vi "Initialize Weather Station.vi"(8 "error in (no error)":errorcluster) -> (0 "error out":errorcluster, 3 "file refnum":refnum<file>, 5 "Weather Data":T1)   [LabVIEW 2010]
doc: "This VI is a part of the Weather Station project. The weather data cluster is created, and a text file (Weather.txt) is created. A header representing the weather data cluster is written to the file.\n\nInputs: Error In\nOutputs: File Refnum, Weather Data Cluster, Error Out"
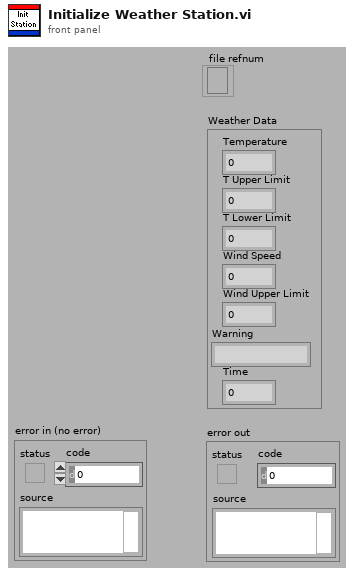
[diagram p1: front panel]
types:
  T1 = cluster{"Temperature":dbl, "T Upper Limit":dbl, "T Lower Limit":dbl, "Wind Speed":dbl, "Wind Upper Limit":dbl, "Warning":string, "Time":dbl}
  T2 = enum16{"open", "replace", "create", "open or create", "replace or create", "replace or create with confirmation"}
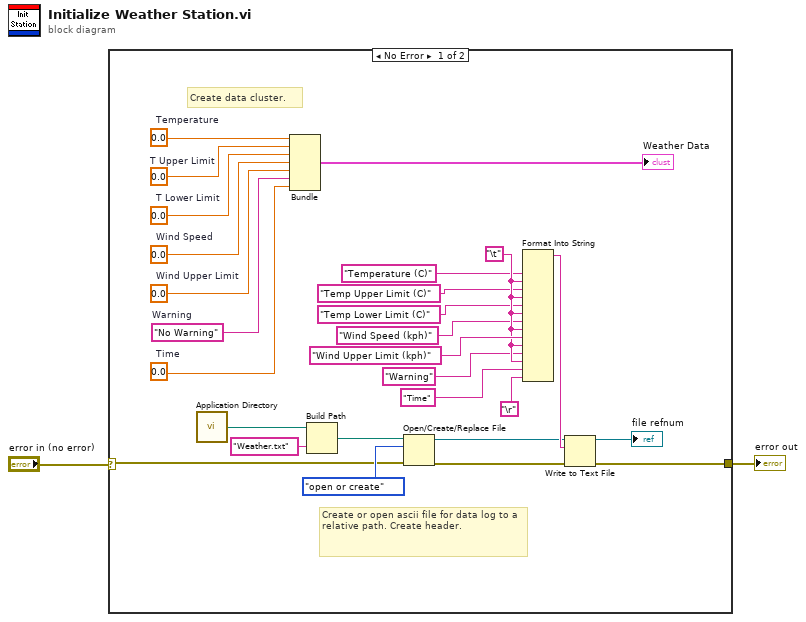
[diagram p0: block diagram]
diagram:
  n1 = case shown="No Error" "error in (no error)" {
    selector: "error in (no error)" -> [w4 w30]
    tunnel: [w28 w30] -> w2
    frame No Error {
      w12 = 0.0  # Time
      w11 = 0.0  # Wind Upper Limit
      w10 = 0.0  # Wind Speed
      w5 = 0.0  # T Lower Limit
      w6 = 0.0  # T Upper Limit
      w7 = 0.0  # Temperature
      w22 = "\t"
      w9 = "No Warning"  # Warning
      # "Create or open ascii file for data log to a relative path. Create header."
      # "Create data cluster."
      n2 = call <vilib>:"Application Directory.vi"() -> ("Application Directory"=w3:path)
      n3 = Bundle("Temperature"=w7, "T Upper Limit"=w6, "T Lower Limit"=w5, "Wind Speed"=w10, "Wind Upper Limit"=w11, "Warning"=w9, "Time"=w12) -> (→"Weather Data":T1)  [unwired: 1 in]
      n4 = Build Path(base path=w3, name or relative path="Weather.txt") -> (appended path=w14:path)
      n5 = Open/Create/Replace File(file path (use dialog)=w14, error in=w4, operation (0:open)=T2."open or create") -> (refnum out=w25:refnum<file>, error out=w27:errorcluster)  [unwired: 3 in, 1 out]
      n6 = Format Into String("Temperature (C)", w22, "Temp Upper Limit (C)", w22, "Temp Lower Limit (C)", w22, "Wind Speed (kph)", w22, "Wind Upper Limit (kph)", w22, "Warning", w22, "Time", "\r") -> (resulting string=w29:string)  [unwired: 3 in, 1 out]
      n7 = Write to Text File(file (use dialog)=w25, text=w29, error in=w27) -> (refnum out=→"file refnum":refnum<file>, error out=w28:errorcluster)  [unwired: 1 in, 1 out]
    }
    frame Error {
    }
  }
  "error out" <- w2
